vi "Init.vi"(8 "error in (no error)":errorcluster, 11 "PDE_2ndOrder_ConstPara":refnum<class "NI_PDE_2ndOrder_ConstPara.lvclass">) -> (0 "error out":errorcluster, 3 "initialized PDE_2ndOrder_ConstPara":refnum<class "NI_PDE_2ndOrder_ConstPara.lvclass">)   [LabVIEW 2017, in "NI_PDE.lvlib" / "NI_PDE_2ndOrder_ConstPara.lvclass"]
uses:
  <vilib>/gmath/pde.llb/PDEClass/PDE_2ndOrder_ConstPara/NI_PDE_2ndOrder_ConstPara.lvclass
  <vilib>/gmath/pde.llb/PDEClass/Class Type.ctl
  <vilib>/gmath/pde.llb/PDEClass/PDE_2ndOrder_ConstPara/NI_PDE_2ndOrder_ConstPara.lvclass/NI_PDE_2ndOrder_ConstPara.ctl
  <vilib>/gmath/pde.llb/PDEClass/NI_PDE.lvclass
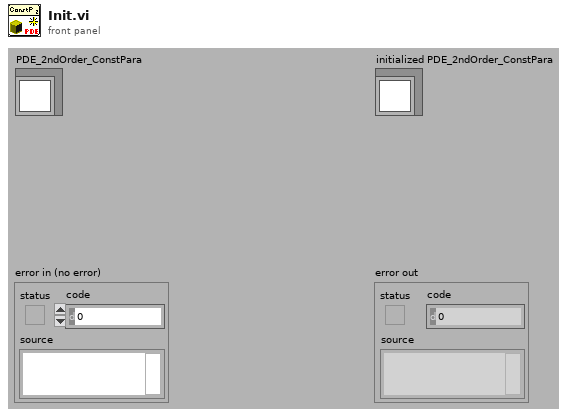
[diagram p1: front panel]
types:
  T1 = typedef "NI_PDE.lvlib/NI_PDE.lvclass/Class Type.ctl" = i32
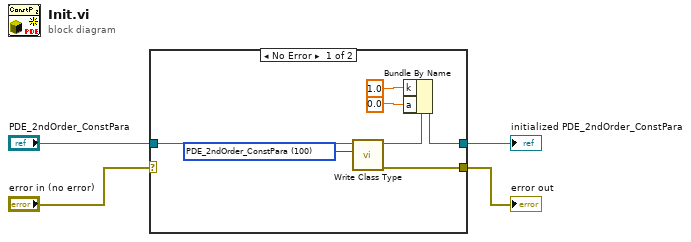
[diagram p0: block diagram]
diagram:
  n1 = case shown="No Error" "error in (no error)" {
    selector: "error in (no error)" -> [_ w13]
    tunnel: "PDE_2ndOrder_ConstPara" -> [w10 w12]
    tunnel: [w8 w12] -> w3
    tunnel: [w7 w13] -> w2
    frame No Error {
      w11 = T1 100 items=["PDE"=0, "PDE_2ndOrder_ConstPara"=100, "PDE_Helmholtz_2D"=112, "PDE_Heat_1D"=121, "PDE_Heat_2D"=122, "PDE_Wave_1D"=131, "PDE_Wave_2D"=132] ("PDE class type")
      n2 = call-dynamic "Write Class Type.vi"("PDE class type"=w11, "PDE.lvclass in"=w10) -> ("error out"=w7:errorcluster, "PDE.lvclass out"=w9:refnum<class "NI_PDE_2ndOrder_ConstPara.lvclass">)  [unwired: 1 in, 7 out]
      n3 = Bundle By Name(cluster=w9, "k"=1.0, "a"=0.0) -> (w8:refnum<class "NI_PDE_2ndOrder_ConstPara.lvclass">)
    }
    frame Error {
    }
  }
  "initialized PDE_2ndOrder_ConstPara" <- w3
  "error out" <- w2
